vi "FTW-CodeGen-AdaptToInputs.vi"(0 "State In":T1 {"Width" format="%dpx"}, 5 "XRef":refnum<vi>, 7 "Term Types":cluster{"Type":variant, "ID":string}[](array[cluster])) -> (4 "State Out":T1 {"Width" format="%dpx"}, 6 "Reply":string[](array[string]))   [LabVIEW 2015, in "FTW-Dataflow-Burrow.xnode"]
uses:
  FTW-Dataflow-Burrow.xnode
  FTW-CodeGen-State.ctl
  framework/FTW-CodeGen-XNodeReplyType.ctl
panel:
  # "Inputs"
  # "Outputs"
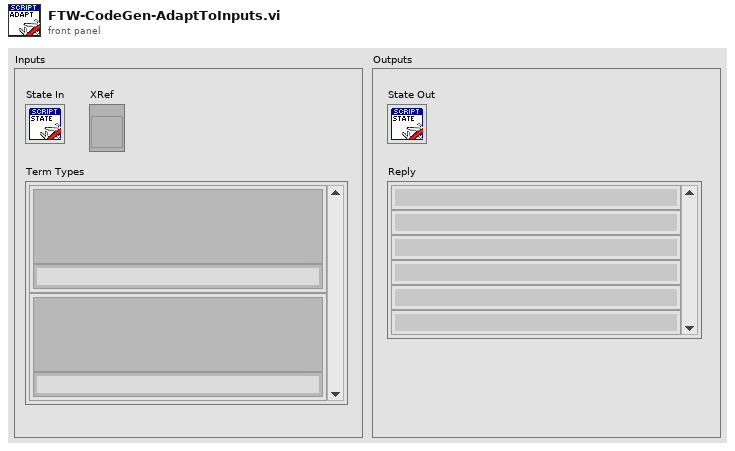
[diagram p1: front panel]
types:
  T1 = typedef "FTW-Dataflow-Burrow.xnode/FTW-CodeGen-State.ctl" = cluster{"InputTerminals":cluster{"Wired?":bool, "ID":string, "DataName":string, "DataColor":u32, "Type":variant}[], "EnableTiming?":bool, "Width":i32}
  T2 = typedef "FTW-CodeGen-XNodeReplyType.ctl" = enum16{"NoReply", "ForceAdaptToInputs", "UpdateTerms", "GenCode", "GenCode+CosmeticUpdate"}
  T3 = cluster{"Wired?":bool, "ID":string, "DataName":string, "DataColor":u32, "Type":variant}[]
  T4 = cluster{"Wired?":bool, "ID":string, "DataName":string, "DataColor":u32, "Type":variant}
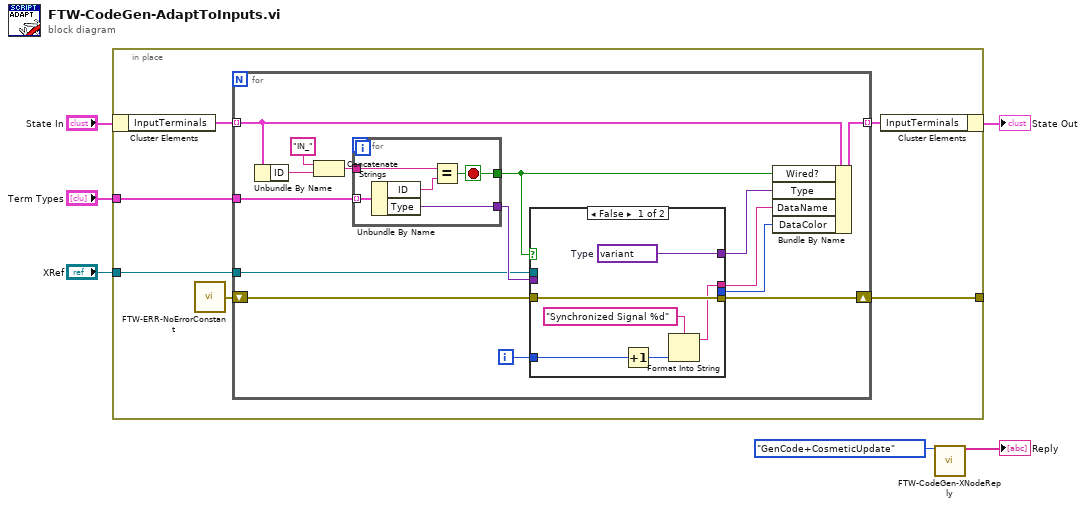
[diagram p0: block diagram]
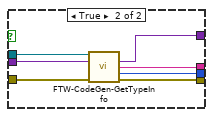
[diagram p2: hidden frame]
diagram:
  n1 = in-place {
    in-place-border: "Term Types" -> [w8]
    in-place-border: [w11] -> _
    in-place-border: "XRef" -> [w7]
    n2 = in-place-cluster #1("State In") -> ("InputTerminals"=w10:T3)
    n3 = call "FTW-ERR-NoErrorConstant.vi"() -> ("no error"=w12:errorcluster)
    n4 = for {
      shift-right: [w27] -> w11
      shift-left: w12 -> [w19]
      tunnel: w10 -> [w25] mode=indexing
      tunnel: [w26] -> w9 mode=indexing
      tunnel: w8 -> [w22]
      tunnel: w7 -> [w18]
      i -> [w13]
      n5 = Unbundle By Name(w25) -> ("ID"=w23:string)
      n6 = Concatenate Strings("IN_" ("format string"), w23) -> (w21:string)
      n7 = for {
        tunnel: [w45] -> w20
        tunnel: [w44] -> w14
        tunnel: w22 -> [w43] mode=indexing
        tunnel: w21 -> [w41]
        stop <- w44 stop-if-true
        n8 = Unbundle By Name(w43) -> ("ID"=w42:string, "Type"=w45:variant)
        n9 = Equal?(x=w41, y=w42) -> (x = y?=w44:bool)
      }
      n10 = case shown="False" w14 {
        tunnel: [w33 w40] -> w27
        tunnel: w20 -> [_ w39]
        tunnel: w19 -> [w33 w38]
        tunnel: w18 -> [_ w37]
        tunnel: [w29 w36] -> w17
        tunnel: [_ w35] -> w16
        tunnel: [w28 w34] -> w15
        tunnel: w13 -> [w30 _]
        frame False {
          w28 = variant(variant variant)  # Type
          n11 = Increment(x=w30) -> (x+1=w32:i32)
          n12 = Format Into String(format string="Synchronized Signal %d" ("Name"), w32) -> (resulting string=w29:string)  [unwired: 2 in, 1 out]
        }
        frame True {
          n13 = call "FTW-CodeGen-GetTypeInfo.vi"("XRef"=w37, "Type Information In"=w39, "error in"=w38) -> ("Safe Type Information for this Context"=w34:variant, "Data Name"=w36:string, "Data Type Color"=w35:u32, "error out"=w40:errorcluster)  [unwired: 9 in]
        }
      }
      n14 = Bundle By Name(cluster=w25, "Wired?"=w14, "Type"=w15, "DataName"=w17, "DataColor"=w16) -> (w26:T4)
    }
    n15 = in-place-cluster #1("InputTerminals"=w9) -> (→"State Out":T1)
  }
  n16 = call "FTW-CodeGen-XNodeReply.vi"("XNode Reply Type"=FTW-CodeGen-XNodeReplyType."GenCode+CosmeticUpdate") -> ("Reply"=→"Reply":string[])  [unwired: 14 in]
